vi "run_cmd_standard_input.vi"(7 "configuration":T1={"username"="", "password"="", "host"="", "type"=enum."ssh"}, 8 "error in (no error)":errorcluster, 11 "command":string) -> (0 "error out":errorcluster, 3 "standard_output":string)   [LabVIEW 2015, in "lv-bin-plink.lvlib" / "v1.lvlib"]
uses:
  v1.lvlib
  _controls/configuration.ctl
  _controls/type.ctl
  <userlib>/antonio-alexander/lv-bin/public/api/v1/v1.lvlib
  lv-bin-plink.lvlib
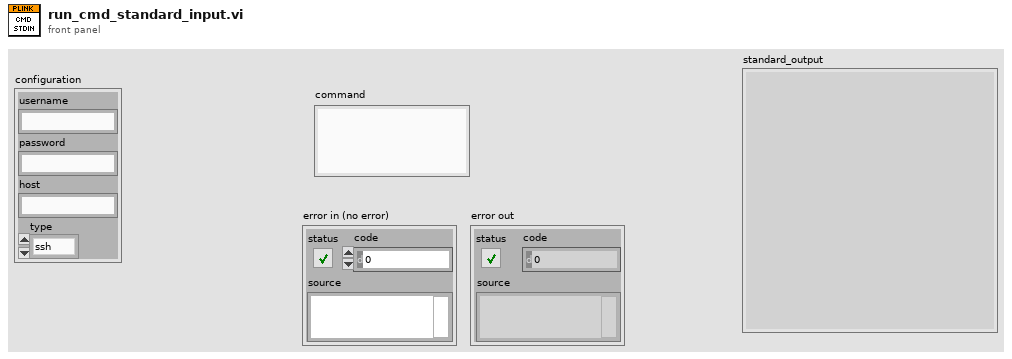
[diagram p1: front panel]
types:
  T1 = typedef "lv-bin-plink.lvlib/v1.lvlib/configuration.ctl" = cluster{"username":string, "password":string, "host":string, "type":T2}
  T2 = typedef "lv-bin-plink.lvlib/v1.lvlib/type.ctl" = enum16{"<type>", "ssh", "telnet", "rlogin", "raw", "serial"}
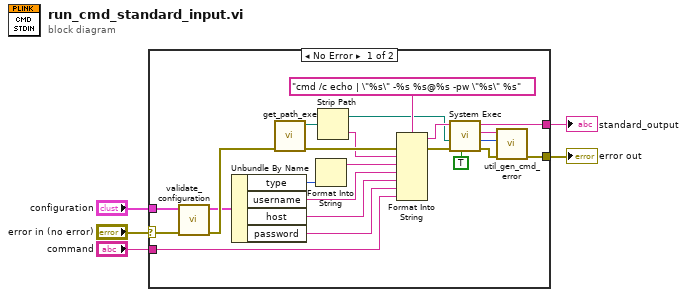
[diagram p0: block diagram]
diagram:
  n1 = case shown="No Error" "error in (no error)" {
    selector: "error in (no error)" -> [w7 w29]
    tunnel: "configuration" -> [w9 _]
    tunnel: [w15 w29] -> w3
    tunnel: [w13 _] -> w2
    tunnel: "command" -> [w11 _]
    frame No Error {
      n2 = call "validate_configuration.vi"("error in (no error)"=w7, "configuration in"=w9) -> ("error out"=w28:errorcluster, "configuration out"=w8:T1)  [unwired: 8 in]
      n3 = Unbundle By Name(w8) -> ("type"=w20:T2, "username"=w18:string, "host"=w17:string, "password"=w16:string)
      n4 = call "get_path_exe.vi"("error in (no error)"=w28) -> ("error out"=w21:errorcluster, "plink"=w12:path)  [unwired: 9 in]
      n5 = Format Into String(w20) -> (resulting string=w19:string)  [unwired: 3 in, 1 out]
      n6 = Strip Path(path=w12) -> (stripped path=w14:path, name=w10:string)
      n7 = Format Into String(format string="cmd /c echo | \"%s\" -%s %s@%s -pw \"%s\" %s", error in=w21, w10, w19, w18, w17, w16, w11) -> (resulting string=w26:string, error out=w25:errorcluster)  [unwired: 1 in]
      n8 = call <vilib>:"System Exec.vi"("run minimized? (F)"=TRUE, "error in (no error)"=w25, "working directory"=w14, "command line"=w26) -> ("error out"=w23:errorcluster, "return code"=w6:i32, "standard error"=w24:string, "standard output"=w13:string)  [unwired: 4 in]
      n9 = call <userlib>:"util_gen_cmd_error.vi"("error in (no error)"=w23, "return_code"=w6, "standard_error"=w24) -> ("error out"=w15:errorcluster)  [unwired: 8 in]
    }
    frame Error {
    }
  }
  "error out" <- w3
  "standard_output" <- w2
